vi "Write Additional Send Headers.vi"(8 "error in (no error)":errorcluster, 10 "Additional Send Headers":T1[](array[typedef]), 11 "Websocket Handler in":refnum<class "Websocket Handler.lvclass">) -> (0 "error out":errorcluster, 3 "Websocket Handler out":refnum<class "Websocket Handler.lvclass">)   [LabVIEW 2020, in "wamplv.lvlib" / "Websocket Handler.lvclass"]
uses:
  Websocket Handler.lvclass
  <vilib>/MediaMongrels Ltd/WebSockets/WebSockets/WebSocket/Headers.ctl
  <vilib>/MediaMongrels Ltd/WebSockets/WebSockets/WebSocket/WebSocket.lvclass
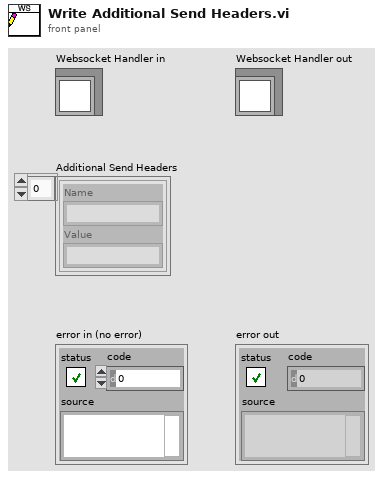
[diagram p1: front panel]
types:
  T1 = typedef "WebSockets.lvlib/WebSocket.lvclass/Headers.ctl" = cluster{"Name":string, "Value":string}
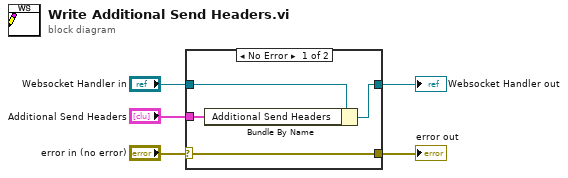
[diagram p0: block diagram]
diagram:
  n1 = case shown="No Error" "error in (no error)" {
    selector: "error in (no error)" -> [w9 w10]
    tunnel: [w9 w10] -> w4
    tunnel: [w7 w11] -> w2
    tunnel: "Websocket Handler in" -> [w8 w11]
    tunnel: "Additional Send Headers" -> [w6 _]
    frame No Error {
      n2 = Bundle By Name(cluster=w8, "Additional Send Headers"=w6) -> (w7:refnum<class "Websocket Handler.lvclass">)
    }
    frame Error {
    }
  }
  "error out" <- w4
  "Websocket Handler out" <- w2
